vi "ColorComponentGenerator.vi"(1 "Component definition":T1={"First color"=0, "Last color"=0, "Middle color"=0, "Middle #"=2} {"Middle #" min=2 max=252}) -> (0 "Component array":u8[](array[numeric]))   [LabVIEW 2019]
doc: "Component Generator.vi is a subVI called by Color Table Generator.vi.\n\nThis VI calculates a range of colors based on initial, middle and final colors. The middle color can be specified at any location within the array. It doesn't have to be the middle index of the array."
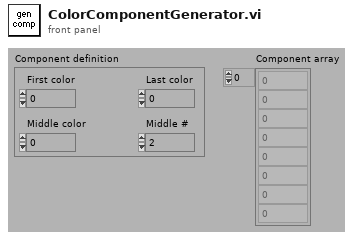
[diagram p1: front panel]
types:
  T1 = cluster{"First color":u8, "Last color":u8, "Middle color":u8, "Middle #":u8}
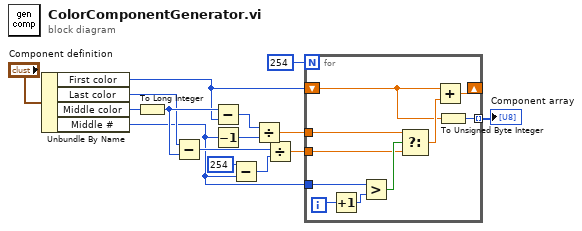
[diagram p0: block diagram]
diagram:
  n1 = Unbundle By Name("Component definition") -> ("First color"=w4:u8, "Last color"=w3:u8, "Middle color"=w1:u8, "Middle #"=w2:u8)
  n2 = To Long Integer(number=w1) -> (32bit integer=w8:i32)
  n3 = Subtract(x=w3, y=w8) -> (x-y=w6:i32)
  n4 = Subtract(x=w8, y=w4) -> (x-y=w7:i32)
  n5 = Decrement(x=w2) -> (x-1=w14:u8)
  n6 = Subtract(x=u8 254, y=w2) -> (x-y=w12:u8)
  n7 = Divide(x=w7, y=w14) -> (x/y=w11:dbl)
  n8 = Divide(x=w6, y=w12) -> (x/y=w10:dbl)
  n9 = for {
    N: 254 -> [_]
    tunnel: w2 -> [w25]
    shift-right: [w18] -> _
    shift-left: w4 -> [w20]
    tunnel: w11 -> [w22]
    tunnel: w10 -> [w21]
    tunnel: [w19] -> w9 mode=indexing
    i -> [w17]
    n10 = Increment(x=w17) -> (x+1=w16:i32)
    n11 = Greater?(x=w25, y=w16) -> (0:w24:bool)
    n12 = Select(t=w22, s=w24, f=w21) -> (s? t:f=w23:dbl)
    n13 = Add(x=w20, y=w23) -> (x+y=w18:dbl)
    n14 = To Unsigned Byte Integer(number=w20) -> (unsigned 8bit integer=w19:u8)
  }
  "Component array" <- w9
